vi "Find Packed Library Classes.vi"(8 "error in (no error)":errorcluster, 10 "packed library path":path, 11 "Component Loader in":refnum<class "Component Loader.lvclass">) -> (0 "error out":errorcluster, 2 "class paths":path[](array[path]), 3 "Component Loader out":refnum<class "Component Loader.lvclass">)   [LabVIEW 2017, in "Data Sharing Framework Core.lvlib" / "Data Sharing Framework Engine.lvlib" / "Component Loader.lvclass"]
uses:
  Component Loader.lvclass
  <vilib>/Utility/LVLibp/NI_PackedLibraryUtility.lvlib
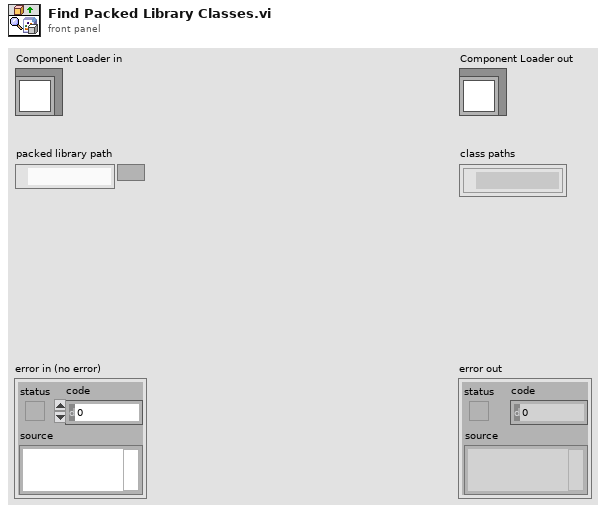
[diagram p1: front panel]
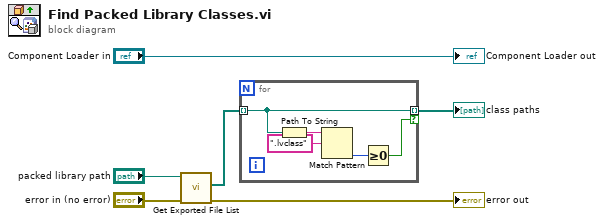
[diagram p0: block diagram]
diagram:
  n1 = call <vilib>:"Get Exported File List.vi"("error in (no error)"="error in (no error)", "packed library path"="packed library path") -> ("error out"=→"error out":errorcluster, "paths"=w2:path[])  [unwired: 7 in, 1 out]
  n2 = for {
    tunnel: w2 -> [w9] mode=indexing
    tunnel: [w9] -> w4 mode=indexing if=w7
    n3 = Path To String(path=w9) -> (string=w10:string)
    n4 = Match Pattern(string=w10, regular expression=".lvclass") -> (offset past match=w8:i32)  [unwired: 1 in, 3 out]
    n5 = Greater Or Equal To 0?(x=w8) -> (x >= 0?=w7:bool)
  }
  "class paths" <- w4
  "Component Loader out" <- "Component Loader in"
